vi "Read StepCount.vi"(8 "error in (no error)":errorcluster, 11 "TestDetailedResult in":refnum<class "TestDetailedResult.lvclass">) -> (0 "error out":errorcluster, 2 "StepCount":u32, 3 "TestDetailedResult out":refnum<class "TestDetailedResult.lvclass">)   [LabVIEW 2019, in "TestEngine.lvlib" / "TestDetailedResult.lvclass"]
uses:
  TestDetailedResult.lvclass
  TestDetailedResult.lvclass/TestDetailedResult.ctl
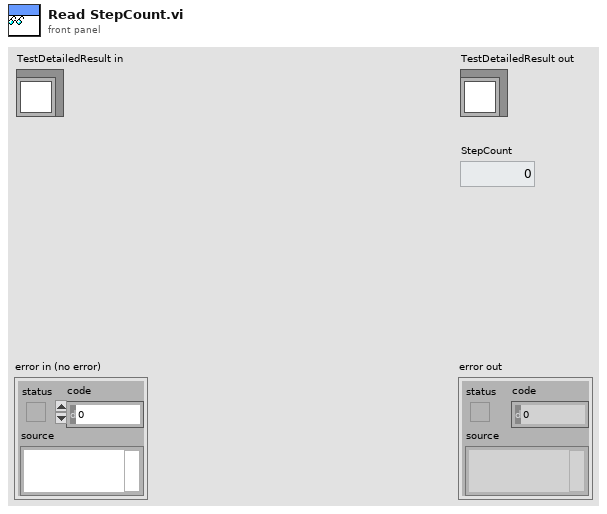
[diagram p1: front panel]
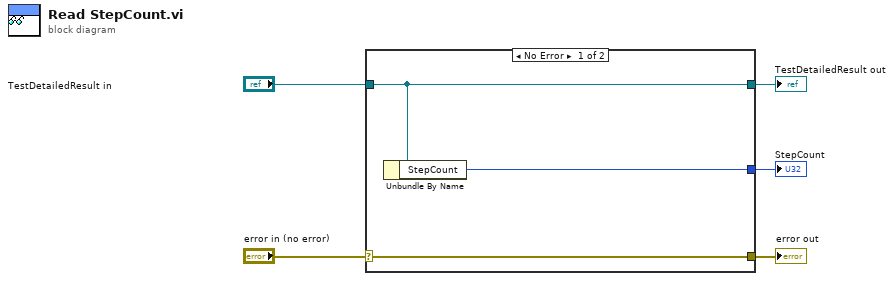
[diagram p0: block diagram]
diagram:
  n1 = case shown="No Error" "error in (no error)" {
    selector: "error in (no error)" -> [w8 w9]
    tunnel: [w8 w9] -> w4
    tunnel: [w7 w10] -> w2
    tunnel: "TestDetailedResult in" -> [w7 w10]
    tunnel: [w6 _] -> w1
    frame No Error {
      n2 = Unbundle By Name(w7) -> ("StepCount"=w6:u32)
    }
    frame Error {
    }
  }
  "error out" <- w4
  "TestDetailedResult out" <- w2
  "StepCount" <- w1
